vi "DriveGetYaw.vi"() -> (3 "Yaw":dbl)   [LabVIEW 2023]
doc: "Put global variable Gyro Z into Yaw to use in other VI's\n\nOutputs:\n -- Yaw -- Double -- Yaw of robot (rotation) --"
uses:
  DriveGlobal.vi
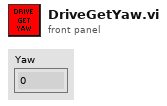
[diagram p1: front panel]
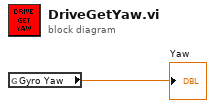
[diagram p0: block diagram]
diagram:
  n1 = global read "DriveGlobal.vi" "Gyro Yaw"() -> (→"Yaw":dbl)
